vi "X test.vi"() -> ()   [LabVIEW 2014]
uses:
  <vilib>/rvi/Emulation/niFpgaGetClockAttributes.vi
  <vilib>/rvi/Emulation/niFpgaSctlEmulationGetInTimedLoop.vi
  <vilib>/rvi/Emulation/niFpgaEmulationReportErrorSimple.vi
  <vilib>/rvi/eio/common/nirviEmuTemplateMethod_errors.vi
  <vilib>/rvi/Emulation/niFpgaCriticalErrorInLSC.vi
  <vilib>/eio/EIONode/EIONode.xnode
panel:
  in  "Count(mSec)":u32=40
  in  "stop":bool
  in  "segment":i16
  out "Waveform Chart":i16(graph)
  out "Connector0/AI2":i16
  in  "x num":i16
  in  "x offset":i16
  in  "step size /1.5nm":i16
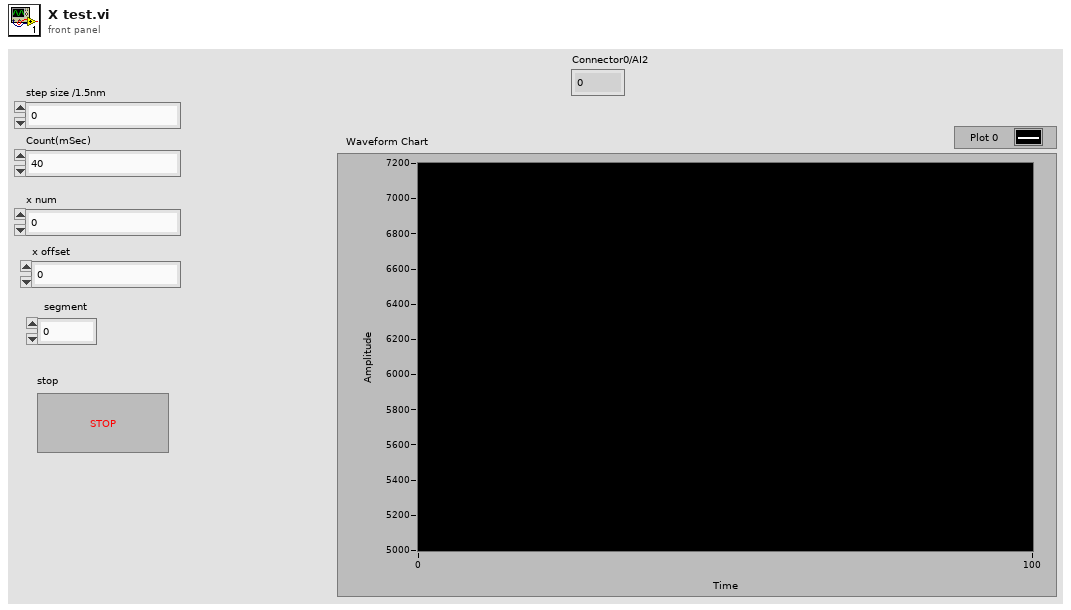
[diagram p1: front panel]
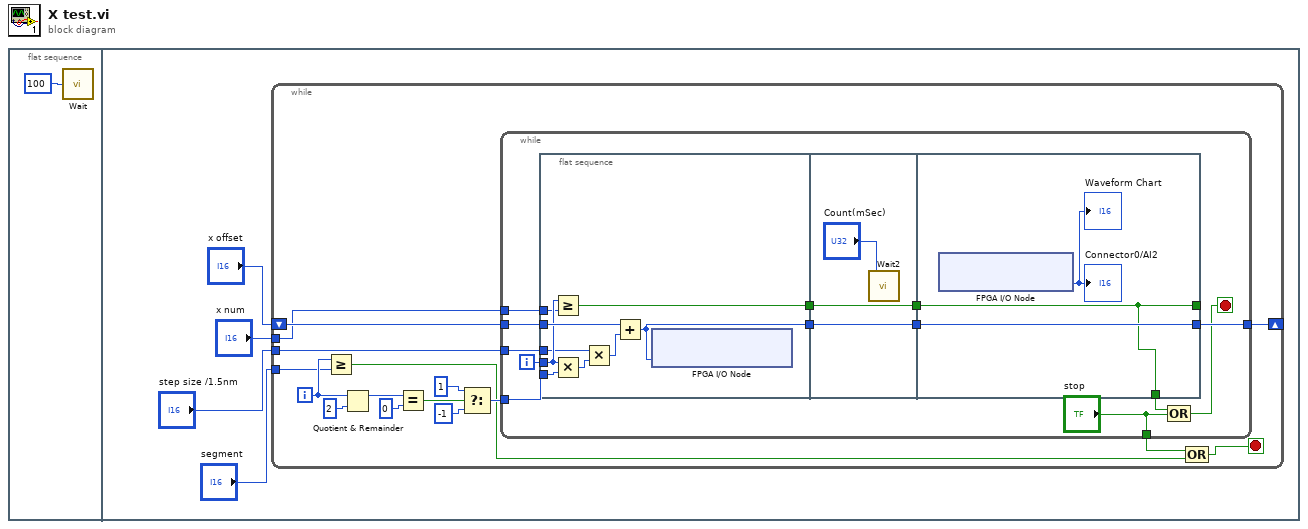
[diagram p0: block diagram]
diagram:
  n1 = flat-sequence {
    frame #0 {
      n2 = call "Wait"("Count(mSec)"=u32 100) -> ()  [unwired: 1 out]
    }
    frame #1 {
      n3 = while {
        tunnel: "step size /1.5nm" -> [w20]
        tunnel: "x num" -> [w12]
        shift-right: [w11] -> _
        shift-left: "x offset" -> [w21]
        tunnel: "segment" -> [w9]
        i -> [w10]
        stop <- w6 stop-if-true
        n4 = Greater Or Equal?(x=w10, y=w9) -> (x >= y?=w7:bool)
        n5 = Quotient & Remainder(x=w10, y=2) -> (x-y*floor(x/y)=w18:i32)  [unwired: 1 out]
        n6 = Equal?(x=w18, y=0) -> (x = y?=w16:bool)
        n7 = Select(t=i16 1, s=w16, f=i16 -1) -> (s? t:f=w13:i16)
        n8 = while {
          tunnel: w20 -> [w33]
          tunnel: w13 -> [w32]
          tunnel: w12 -> [w30]
          tunnel: w21 -> [w34]
          tunnel: [w29] -> w11
          tunnel: ["stop"] -> w8
          i -> [w31]
          stop <- w23 stop-if-true
          n9 = flat-sequence {
            tunnel: w34 -> [w43]
            tunnel: w33 -> [w35]
            tunnel: w32 -> [w41]
            tunnel: w31 -> [w39]
            tunnel: w30 -> [w38]
            tunnel: [w37] -> w28
            tunnel: [w36] -> w27
            tunnel: w28 -> [w46]
            tunnel: w27 -> [w45]
            tunnel: [w46] -> w26
            tunnel: [w45] -> w25
            tunnel: [w49] -> w29
            tunnel: [w47] -> _
            tunnel: w26 -> [w47]
            tunnel: w25 -> [w49]
            tunnel: [w47] -> w24
            frame #0 {
              n10 = Greater Or Equal?(x=w39, y=w38) -> (x >= y?=w37:bool)
              n11 = Multiply(x=w39, y=w41) -> (x*y=w40:i32)
              n12 = Multiply(x=w35, y=w40) -> (x*y=w42:i32)
              n13 = Add(x=w43, y=w42) -> (x+y=w36:i32)
              n14 = xnode "FPGA I/O Node"("Connector0/AO2"=w36) -> ()  [unwired: 1 in, 1 out]
            }
            frame #1 {
              n15 = call "Wait2"("Count(mSec)"="Count(mSec)") -> ()  [unwired: 1 out]
            }
            frame #2 {
              n16 = xnode "FPGA I/O Node"() -> ("Connector0/AI2"=→"Connector0/AI2" →"Waveform Chart":i16)  [unwired: 1 in, 1 out]
            }
          }
          n17 = Compound Arithmetic op=OR(w24, "stop") -> (w23:bool)
        }
        n18 = Compound Arithmetic op=OR(w8, w7) -> (w6:bool)
      }
    }
  }
